vi "Init.vi"(3 "Container State":T4, 4 "Previous State":variant, 5 "Previous Version":T3) -> (2 "Current State":T1={"logTable"=refnum, "max items"=500, "displaydata"=[], "data"=[], "Auto Scroll"=TRUE, "current item"=500, "col headers"=[], "Add to Top"=TRUE, "Auto resize"=TRUE, "col size"=[], "filters"=[], "color cells"=[]})   [LabVIEW 2013, in "UI-DisplayTable(dev).xctl"]
uses:
  UI-DisplayTable(dev).xctl
  State.ctl
  Support/DEF-Filter.ctl
  <vilib>/_xctls/Container State.ctl
  <vilib>/_xctls/Version.ctl
  <vilib>/_xctls/XControlSupport.lvlib
panel:
  in  "Default Indicator State":T1={"logTable"=refnum, "max items"=500, "displaydata"=[], "data"=[], "Auto Scroll"=TRUE, "current item"=500, "col headers"=[], "Add to Top"=TRUE, "Auto resize"=TRUE, "col size"=[], "filters"=[], "color cells"=[]}
  in  "Default Control State":T1={"logTable"=refnum, "max items"=500, "displaydata"=[], "data"=[], "Auto Scroll"=TRUE, "current item"=500, "col headers"=[], "Add to Top"=TRUE, "Auto resize"=TRUE, "col size"=[], "filters"=[], "color cells"=[]}
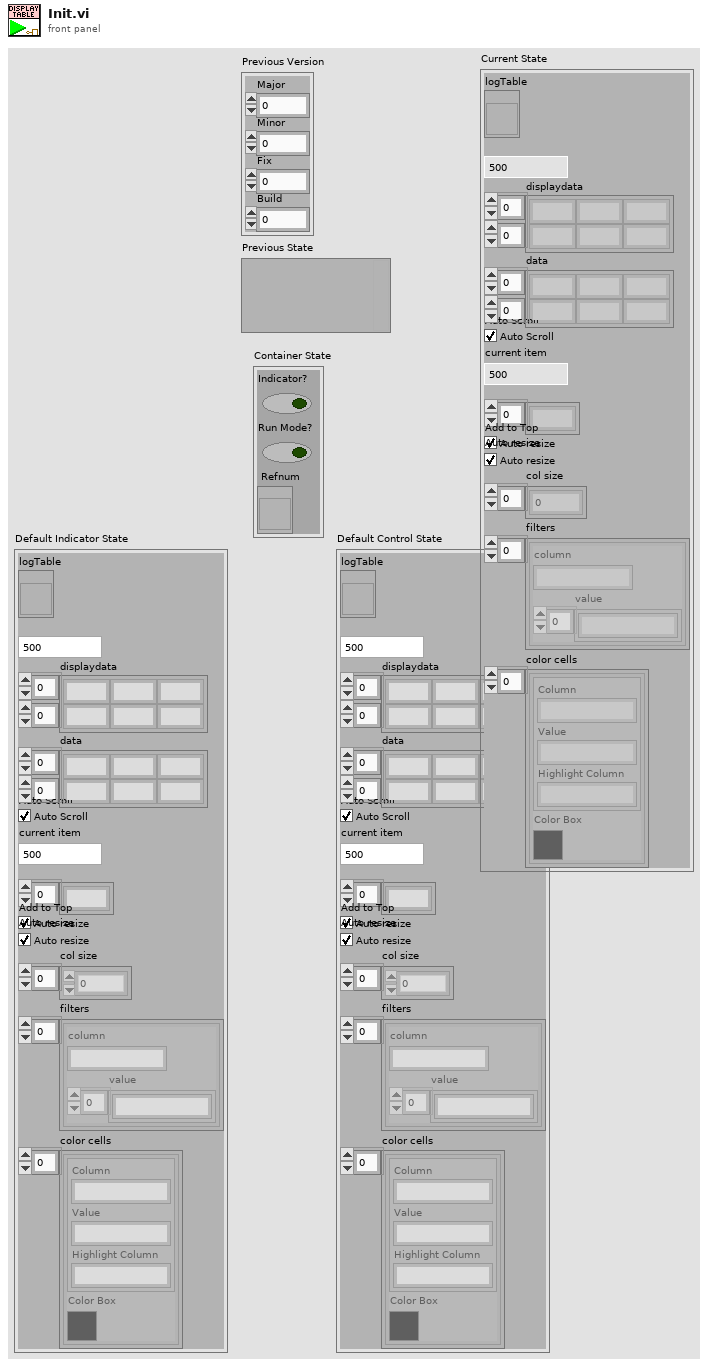
[diagram p1: front panel]
types:
  T1 = typedef "UI-DisplayTable(dev).xctl/State.ctl" = cluster{"logTable":refnum<vi>, "max items":i32, "displaydata":string[][], "data":string[][], "Auto Scroll":bool, "current item":i32, "col headers":string[], "Add to Top":bool, "Auto resize":bool, "col size":i32[], "filters":T2[], "color cells":cluster{"color cell":cluster{"Column":string, "Value":string, "Highlight Column":string}, "Color Box":u32}[]}
  T2 = typedef "UI-DisplayTable(dev).xctl/DEF-Filter.ctl" = cluster{"column":string, "value":string[]}
  T3 = typedef "XControlSupport.lvlib/Version.ctl" = cluster{"Major":u16, "Minor":u16, "Fix":u16, "Build":u16}
  T4 = typedef "XControlSupport.lvlib/Container State.ctl" = cluster{"Indicator?":bool, "Run Mode?":bool, " Refnum":refnum<vi>}
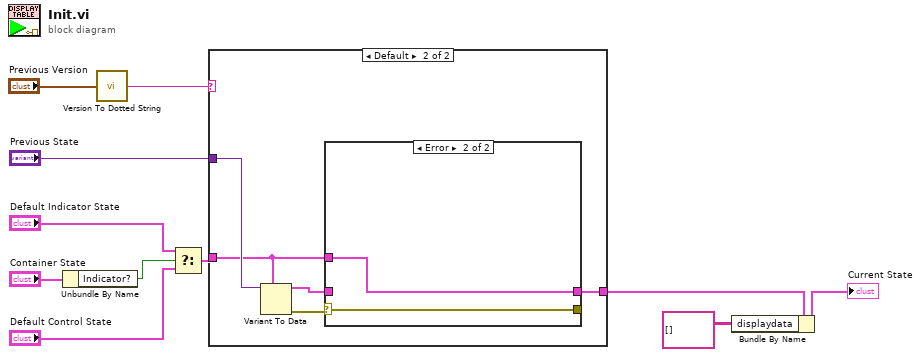
[diagram p0: block diagram]
diagram:
  n1 = Unbundle By Name("Container State") -> ("Indicator?"=w6:bool)
  n2 = call <vilib>:"Version To Dotted String.vi"("Version"="Previous Version") -> ("String Version"=w3:string)
  n3 = Select(t="Default Indicator State", s=w6, f="Default Control State") -> (s? t:f=w5:T1)
  n4 = case shown="Default" w3 {
    tunnel: "Previous State" -> [_ w17]
    tunnel: [w12 w13] -> w10
    tunnel: w5 -> [w12 w14]
    frame "0.0.0.0" {
      # "Just created, use default state"
    }
    frame Default {
      n5 = Variant To Data(type=w14, Variant=w17) -> (data=w15:T1, error out=w16:errorcluster)  [unwired: 1 in]
      n6 = case shown="Error" w16 {
        selector: w16 -> [w19 w20]
        tunnel: w15 -> [w18 _]
        tunnel: [w18 w21] -> w13
        tunnel: w14 -> [_ w21]
        tunnel: [w19 w20] -> _
        frame No Error {
        }
        frame Error {
        }
      }
    }
  }
  n7 = Bundle By Name(cluster=w10, "displaydata"=string[][] []) -> (→"Current State":T1)
